vi "Get Device State.vi"(0 "Interface_object in":refnum<class "Lamp.lvclass">, 5 "error in (no error)":errorcluster) -> (14 "Interface_object out":refnum<class "Lamp.lvclass">, 17 "Device State":bool, 19 "error out":errorcluster)   [LabVIEW 2018, in "Lamp.lvclass"]
uses:
  Lamp.lvclass
  Lamp.lvclass/Lamp.ctl
  Get Is Turned ON.vi
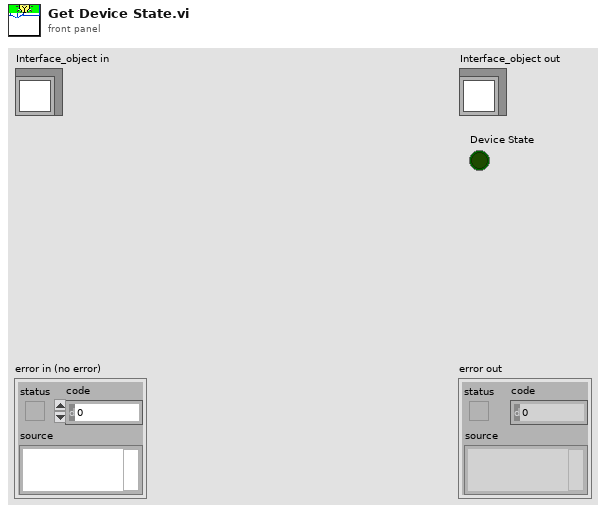
[diagram p1: front panel]
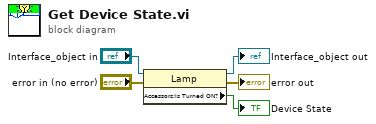
[diagram p0: block diagram]
diagram:
  n1 = property class="Lamp"(reference="Interface_object in", error in="error in (no error)") -> (reference out=→"Interface_object out":refnum<class "Lamp.lvclass">, error out=→"error out":errorcluster, "Accessors:Is Turned ON?"=→"Device State":bool)
